vi "Translate_test.vi"(0 "Speed":i16, 11 "Turn":i16) -> (4 "Right Motor Speed":i16, 15 "Left Motor Speed":i16)   [LabVIEW 2009]
doc: "This VI takes in Speed and Turn values and converts them into wheel speeds.\nNOTE : Turn value of 0 indicates that the robot will go straight"
panel:
  in  "Wheel Diameter 2":dbl=0.4191 caption="Wheel Diameter=r(m)"
  out "Global wl":dbl
  out "Global wr":dbl
  out "wl":dbl caption="Left wheel angular velocity=wl(R/s)"
  out "wr":dbl caption="Right wheel angular velocity=wr(R/s)"
  in  "Wheel Diameter":dbl=0.21 caption="Wheel Radius=r(m)"
  in  "Distance Between wheels":dbl=0.6096 caption="Distance between wheels=L(m)"
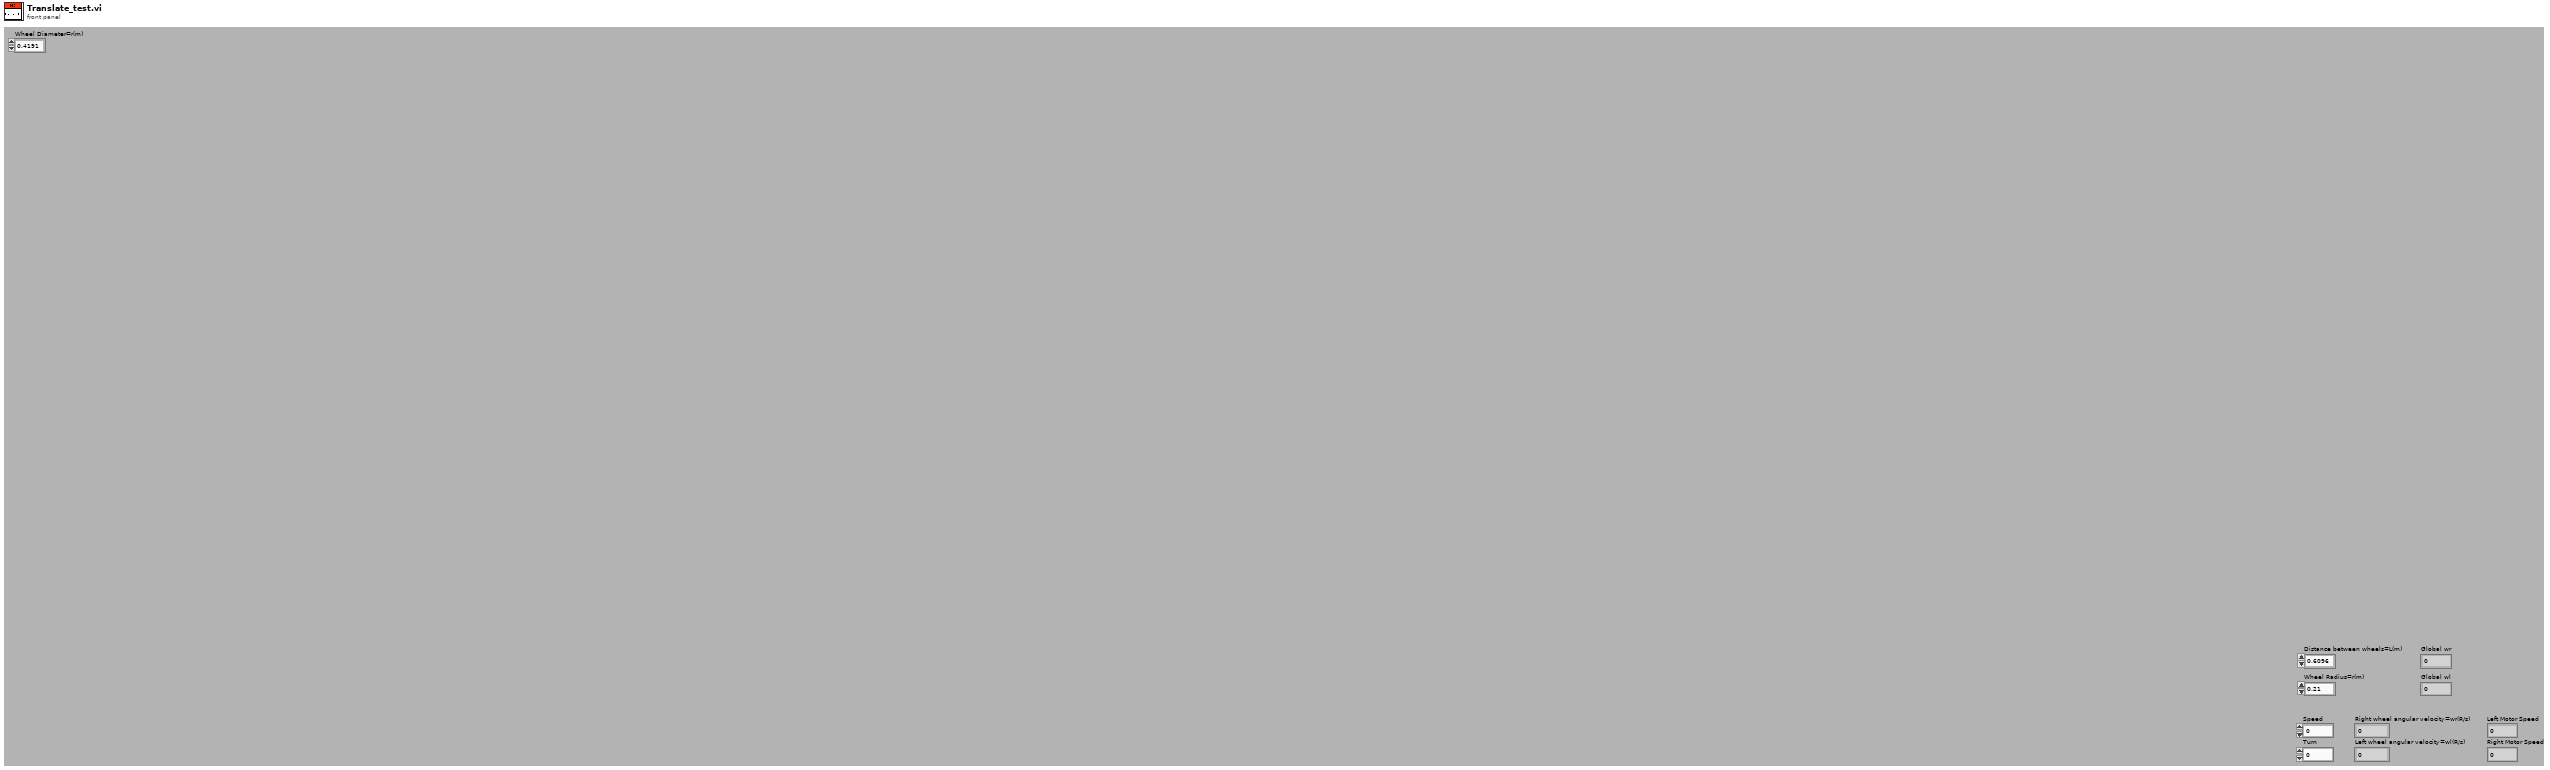
[diagram p1: front panel]
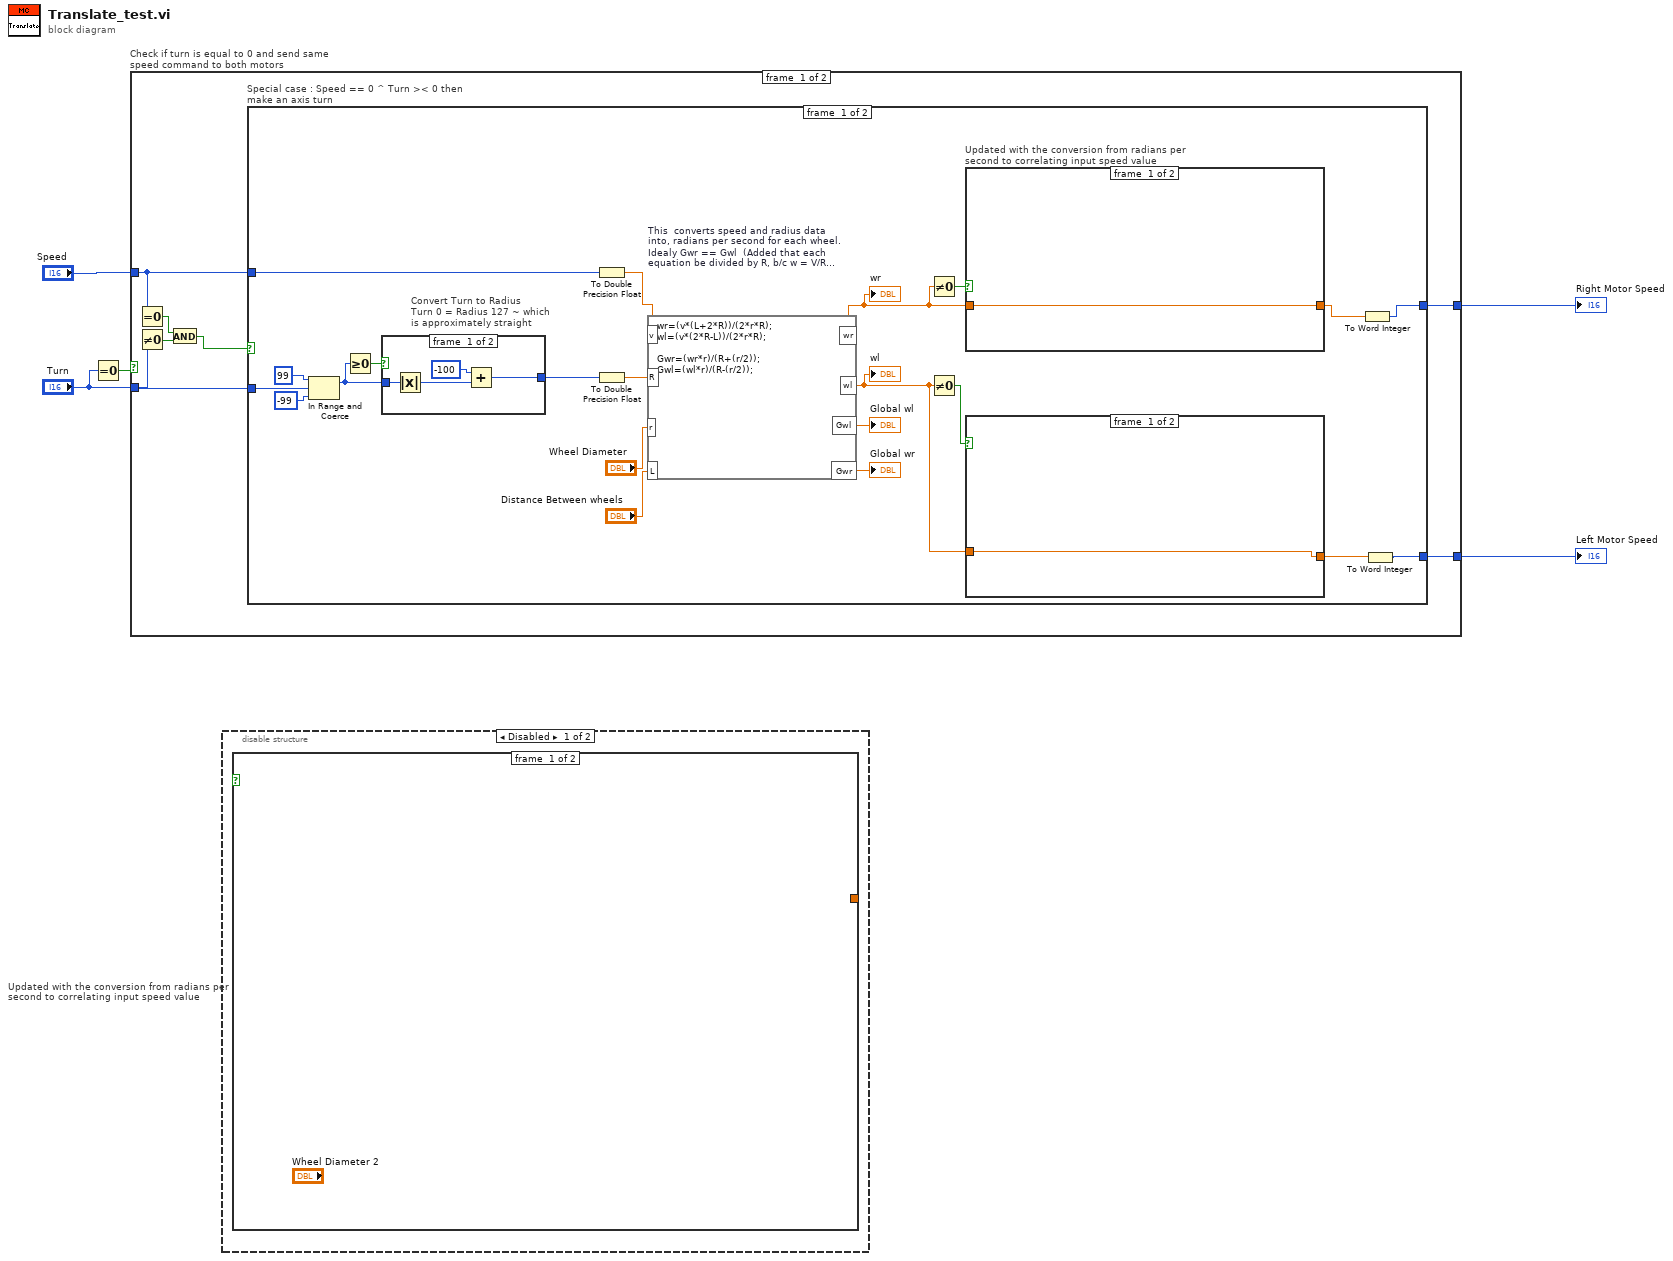
[diagram p0: block diagram]
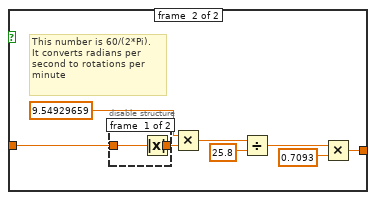
[diagram p2: hidden frame]
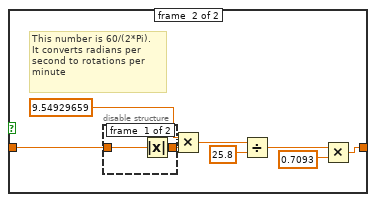
[diagram p4: hidden frame]
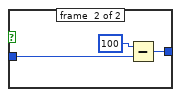
[diagram p6: hidden frame]
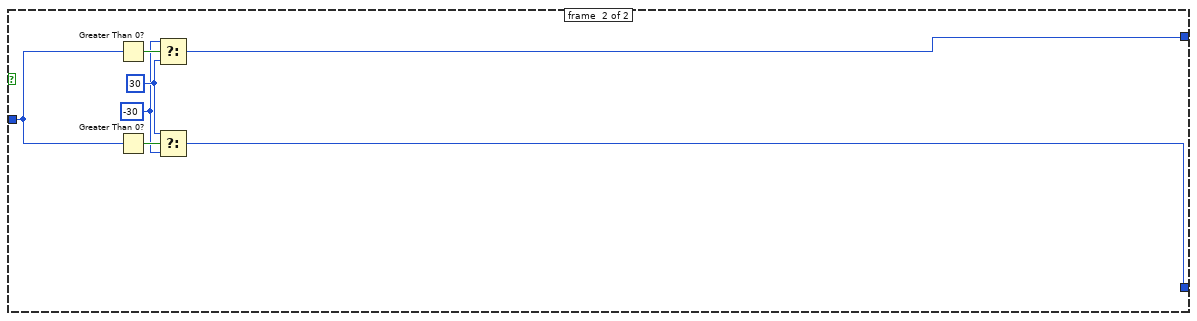
[diagram p7: hidden frame]
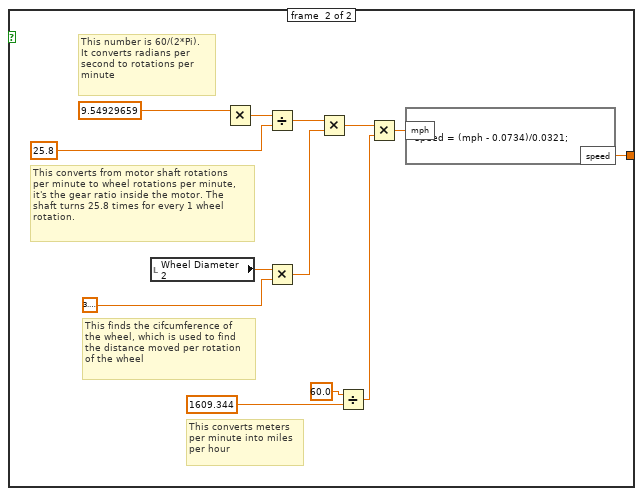
[diagram p9: hidden frame]
diagram:
  n1 = Equal To 0?(x="Turn") -> (x = 0?=w4:bool)
  n2 = case "Check if turn is equal to 0 and send same speed command to both motors" shown="False" w4 {
    tunnel: "Turn" -> [w8 _]
    tunnel: "Speed" -> [w10 w72]
    tunnel: [w12 w72] -> w2
    tunnel: [w11 w72] -> w1
    frame #0 {
      n3 = Equal To 0?(x=w10) -> (x = 0?=w9:bool)
      n4 = Not Equal To 0?(x=w8) -> (x != 0?=w6:bool)
      n5 = And(x=w9, y=w6) -> (x .and. y?=w7:bool)
      n6 = case "Special case : Speed == 0 ^ Turn >< 0 then make an axis turn" shown="True" w7 {
        tunnel: w8 -> [w27 w69]
        tunnel: w10 -> [w17 _]
        tunnel: [w15 w66] -> w12
        tunnel: [w13 w65] -> w11
        frame #0 {
          n7 = In Range and Coerce(upper limit=i16 99, x=w27, lower limit=i16 -99) -> (coerced(x)=w24:i16)  [unwired: 1 out]
          n8 = Greater Or Equal To 0?(x=w24) -> (x >= 0?=w28:bool)
          n9 = case "Convert Turn to Radius\nTurn 0 = Radius 127 ~ which\nis approximately straight" shown="True" w28 {
            tunnel: w24 -> [w59 w64]
            tunnel: [w58 w62] -> w23
            frame #0 {
              n10 = Absolute Value(x=w59) -> (abs(x)=w60:i16)
              n11 = Add(x=i16 -100, y=w60) -> (x+y=w58:i16)
            }
            frame #1 {
              n12 = Subtract(x=i16 100, y=w64) -> (x-y=w62:i16)
            }
          }
          n13 = To Double Precision Float(number=w17) -> (double precision float=w18:dbl)
          n14 = To Double Precision Float(number=w23) -> (double precision float=w29:dbl)
          n15 = formula code="wr=(v*(L+2*R))/(2*r*R);\nwl=(v*(2*R-L))/(2*r*R);\n\nGwr=(wr*r)/(R+(r/2));\nGwl=(wl*r)/(R-(r/2));" "This  converts speed and radius data \ninto, radians per second for each wheel.\nIdealy Gwr == Gwl  (Added that each \nequation be divided by R, b/c w = V/R \nand earlier the equations only equated\nto V NOT w.  Also removed r from the\nwr and wl equations (2*r*R) because\nthey were not used when first deriving\nthe required equation for wr and wl)"("v"=w18, "R"=w29, "r"="Wheel Diameter", "L"="Distance Between wheels") -> ("wr"=w21:dbl, "wl"=w19:dbl, "Gwr"=→"Global wr":dbl, "Gwl"=→"Global wl":dbl)
          "wr" <- w21
          "wl" <- w19
          n16 = Not Equal To 0?(x=w21) -> (x != 0?=w22:bool)
          n17 = Not Equal To 0?(x=w19) -> (x != 0?=w20:bool)
          n18 = case "Updated with the conversion from radians per second to correlating input speed value" shown="True" w22 {
            tunnel: w21 -> [w46 w48]
            tunnel: [w46 w47] -> w16
            frame #0 {
            }
            frame #1 {
              # "This number is 60/(2*Pi). \nIt converts radians per \nsecond to rotations per \nminute"
              n19 = disable-structure shown="Enabled" {
                disable-tunnel: [w56 w57] -> w52
                disable-tunnel: w48 -> [w55 w57]
                frame #0 {
                  n20 = Absolute Value(x=w55) -> (abs(x)=w56:dbl)
                }
                frame #1 {
                }
              }
              n21 = Multiply(x=9.54929659, y=w52) -> (x*y=w51:dbl)
              n22 = Divide(x=w51, y=25.8) -> (x/y=w49:dbl)
              n23 = Multiply(x=w49, y=0.7093 ("x")) -> (x*y=w47:dbl)
            }
          }
          n24 = case shown="True" w20 {
            tunnel: w19 -> [w34 w36]
            tunnel: [w34 w35] -> w14
            frame #0 {
            }
            frame #1 {
              # "This number is 60/(2*Pi). \nIt converts radians per \nsecond to rotations per \nminute"
              n25 = disable-structure shown="Enabled" {
                disable-tunnel: [w44 w45] -> w40
                disable-tunnel: w36 -> [w43 w45]
                frame #0 {
                  n26 = Absolute Value(x=w43) -> (abs(x)=w44:dbl)
                }
                frame #1 {
                }
              }
              n27 = Multiply(x=9.54929659, y=w40) -> (x*y=w39:dbl)
              n28 = Divide(x=w39, y=25.8) -> (x/y=w37:dbl)
              n29 = Multiply(x=w37, y=0.7093 ("x")) -> (x*y=w35:dbl)
            }
          }
          n30 = To Word Integer(number=w16) -> (16bit integer=w15:i16)
          n31 = To Word Integer(number=w14) -> (16bit integer=w13:i16)
        }
        frame #1 {
          w68 = i16 30 ("t")
          w67 = i16 -30 ("t")
          n32 = Greater Than 0?(x=w69) -> (x > 0?=w71:bool)
          n33 = Greater Than 0?(x=w69) -> (x > 0?=w70:bool)
          n34 = Select(t=w67, s=w71, f=w68) -> (s? t:f=w66:i16)
          n35 = Select(t=w68, s=w70, f=w67) -> (s? t:f=w65:i16)
        }
      }
    }
    frame #1 {
    }
  }
  "Right Motor Speed" <- w2
  "Left Motor Speed" <- w1
  n36 = disable-structure shown="Disabled" {
    frame #0 {
      n37 = case "Updated with the conversion from radians per second to correlating input speed value" shown="True" {
        selector: _ -> [_ _]
        tunnel: [_ w73] -> _
        frame #0 {
        }
        frame #1 {
          # "This converts meters\nper minute into miles\nper hour"
          # "This finds the cifcumference of\nthe wheel, which is used to find \nthe distance moved per rotation\nof the wheel"
          # "This converts from motor shaft rotations \nper minute to wheel rotations per minute,\nit's the gear ratio inside the motor. The \nshaft turns 25.8 times for every 1 wheel \nrotation."
          # "This number is 60/(2*Pi). \nIt converts radians per \nsecond to rotations per \nminute"
          n38 = local read "Wheel Diameter 2"() -> (w80:dbl)
          n39 = Multiply(x=9.54929659) -> (x*y=w84:dbl)  [unwired: 1 in]
          n40 = Divide(x=w84, y=25.8) -> (x/y=w82:dbl)
          n41 = Multiply(x=w80, y=3.141592653589793) -> (x*y=w79:dbl)
          n42 = Multiply(x=w82, y=w79) -> (x*y=w78:dbl)
          n43 = Divide(x=60.0, y=1609.344) -> (x/y=w75:dbl)
          n44 = Multiply(x=w78, y=w75) -> (x*y=w74:dbl)
          n45 = formula code="speed = (mph - 0.0734)/0.0321;"("mph"=w74) -> ("speed"=w73:dbl)
        }
      }
    }
    frame #1 {
    }
  }
